vi "CreateSourcesNode.vi"(7 "DOM Document":refnum<k20>, 8 "Error In":errorcluster, 11 "Sources":T1[](array[typedef])) -> (0 "Error Out":errorcluster, 3 "Sources Node":refnum<k20>)   [LabVIEW 2013]
uses:
  SourceConfiguration.ctl
  SourceFunction.ctl
  libs/LV-Utilities/LV-Utilities.lvlib
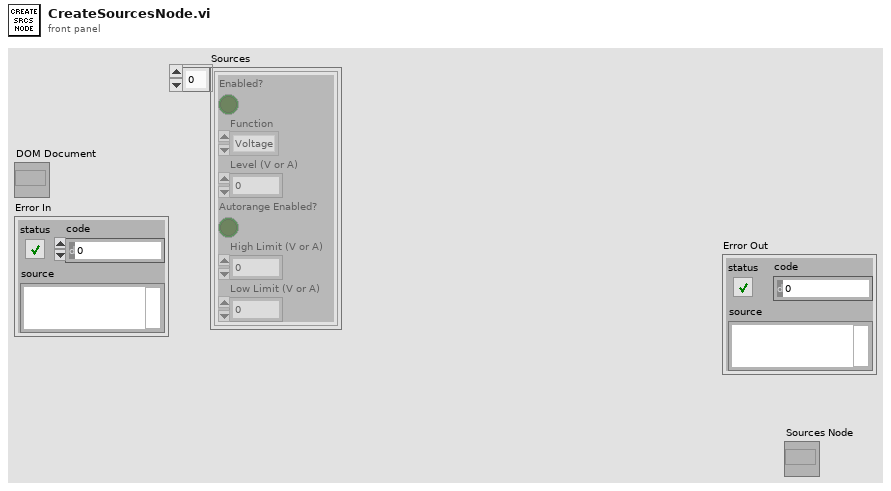
[diagram p1: front panel]
types:
  T1 = typedef "SourceConfiguration.ctl" = cluster{"Enabled?":bool, "Function":T2, "Level (V or A)":dbl, "Autorange Enabled?":bool, "High Limit (V or A)":dbl, "Low Limit (V or A)":dbl}
  T2 = typedef "SourceFunction.ctl" = enum16{"Voltage", "Current"}
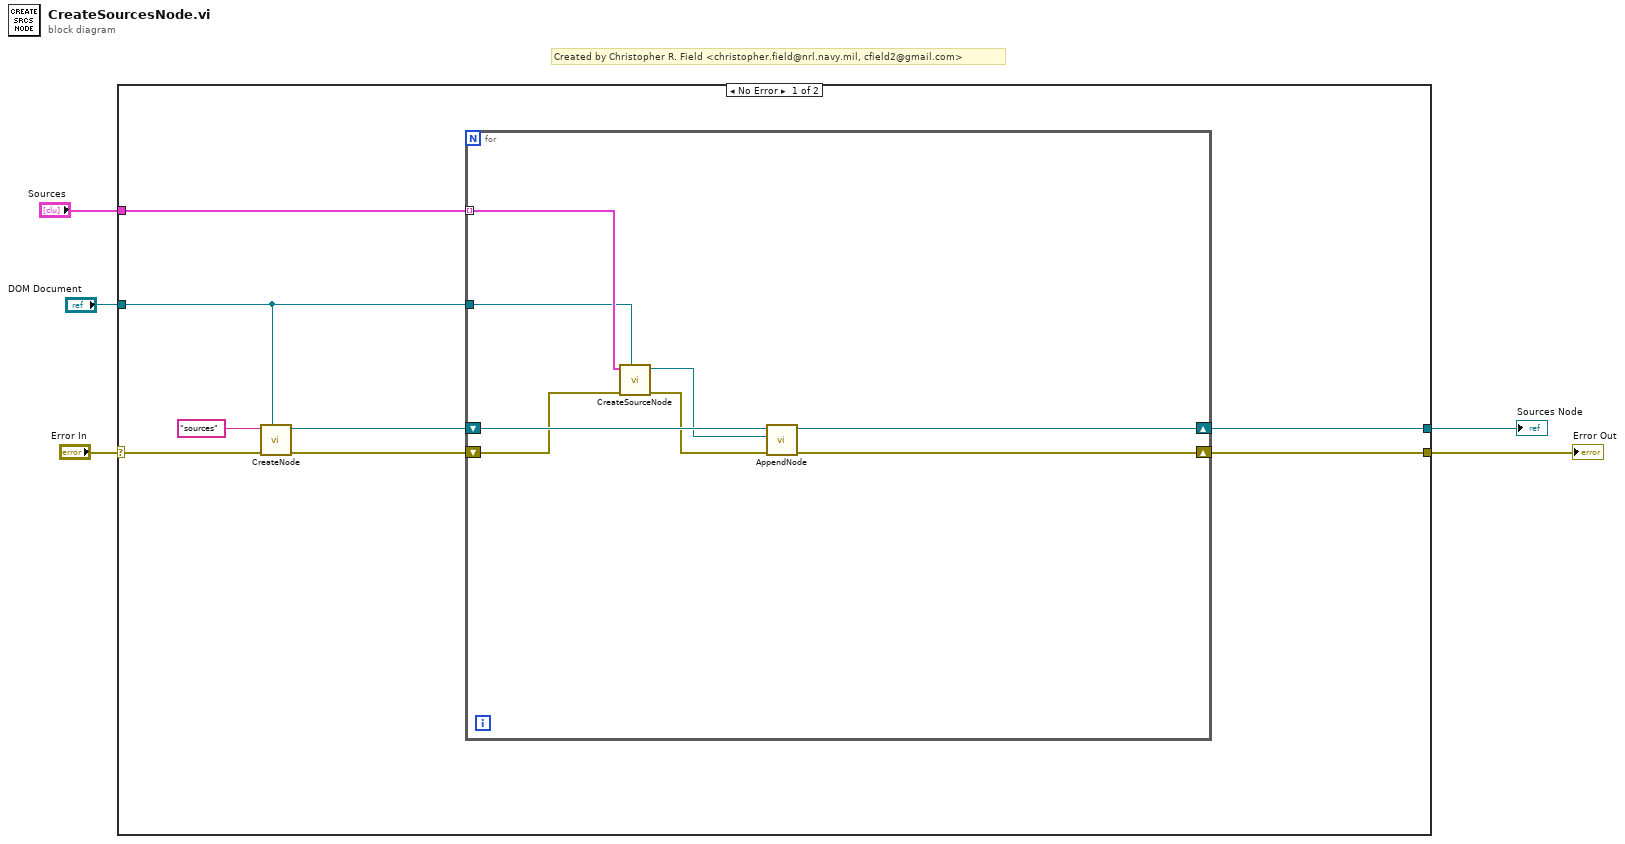
[diagram p0: block diagram]
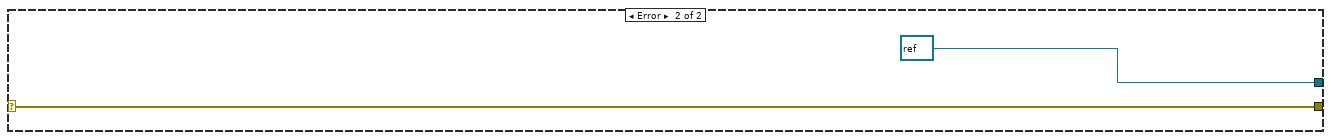
[diagram p2: hidden frame]
diagram:
  # "Created by Christopher R. Field <christopher.field@nrl.navy.mil, cfield2@gmail.com>"
  n1 = case shown="No Error" "Error In" {
    selector: "Error In" -> [w12 w23]
    tunnel: "DOM Document" -> [w6 _]
    tunnel: [w7 w23] -> w3
    tunnel: [w8 refnum<k20> refnum ("DUT Node 2")] -> w2
    tunnel: "Sources" -> [w13 _]
    frame No Error {
      n2 = call "CreateNode.vi"("DOM Document"=w6, "Error In"=w12, "Tag Name"="sources") -> ("Error out"=w9:errorcluster, "Node"=w10:refnum<k20>)  [unwired: 7 in]
      n3 = for {
        tunnel: w13 -> [w18] mode=indexing
        shift-right: [w20] -> w7
        shift-left: w9 -> [w16]
        shift-right: [w19] -> w8
        shift-left: w10 -> [w21]
        tunnel: w6 -> [w17]
        n4 = call "CreateSourceNode.vi"("DOM Document"=w17, "Error In"=w16, "Source Configuration"=w18) -> ("Error Out"=w15:errorcluster, "Source Node"=w14:refnum<k20>)  [unwired: 7 in]
        n5 = call "AppendNode.vi"("Error In"=w15, "Child Node"=w14, "Parent Node In"=w21) -> ("Error Out"=w20:errorcluster, "Parent Node Out"=w19:refnum<k20>)  [unwired: 7 in]
      }
    }
    frame Error {
    }
  }
  "Error Out" <- w3
  "Sources Node" <- w2
